vi "DAQ_DECM Configure and Measure.vi"(0 "DAQmx Tasks In":T1, 2 "Execution Option":T3, 5 "Counter Settings":T4={"Active Edge"=10280, "Duration (s)"=0.1, "Wait Type"=enum."Hardware Timed"} {"Duration (s)" format="%.2p"; "Active Edge" items=["Rising"=10280, "Falling"=10171]}, 7 "Timer - Trigger Settings":T2={"Trigger Type"=enum."No Trigger", "Digital Start Trigger Source"="", "Digital Start Trigger Edge"=10280} {"Digital Start Trigger Edge" items=["Rising"=10280, "Falling"=10171]}, 11 "error in":errorcluster) -> (4 "DAQmx Tasks Out":T1, 6 "Edge Counts":u32, 15 "error out":errorcluster)   [LabVIEW 2021, in "DAQ_Digital Edge Count Measurement.lvlib"]
doc: "Configure, initiate and fetch no of digital events/edges detected from the channel configured.\n\nNOTE: Initialize VI is recommended to create tasks instead of using tasks defined in NI-MAX directly. because initialize takes care of routing the output terminal of Timer task internally to reduce the need for additional PFI line output terminal.\n\nRefer detailed help for more details on hardware timed vs software timed digital edge counting. And use the inputs accordingly."
uses:
  DAQ_Digital Edge Count Measurement.lvlib
  Typedefs/Measurement Settings.ctl
  Typedefs/Wait Type.ctl
  Common/Typedefs/Execution Options - Measure.ctl
  Typedefs/Timer - Trigger Settings.ctl
  Typedefs/DAQmx Tasks.ctl
  <vilib>/DAQmx/read.llb/DAQmx Read (Counter U32 1Chan 1Samp).vi
  <vilib>/DAQmx/configure/trigger.llb/DAQmx Start Trigger (Digital Edge).vi
  <vilib>/DAQmx/miscellaneous.llb/DAQmx Fill In Error Info.vi
  <resource>/objmgr/daqmx.rc
panel:
  # "Inputs"
  # "Outputs"
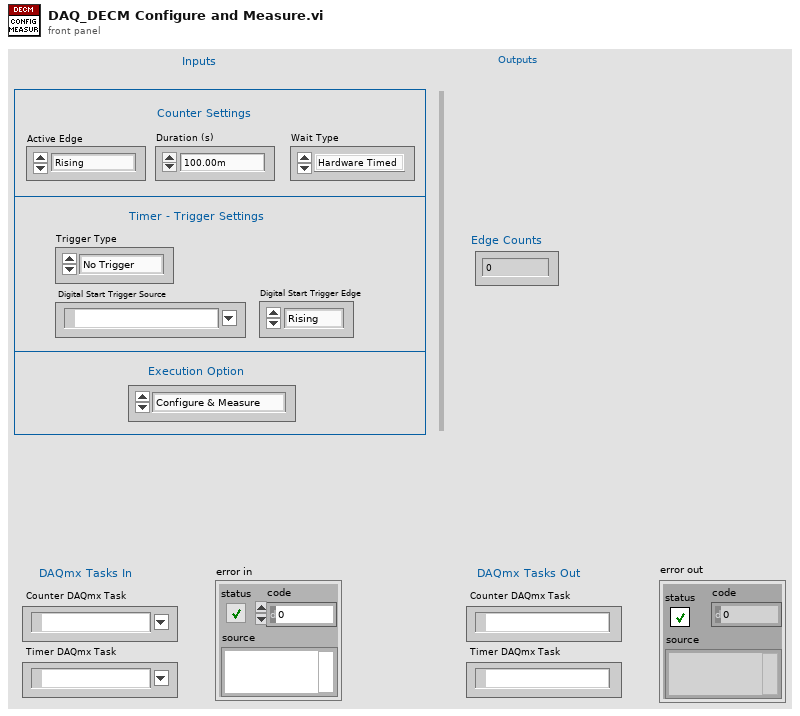
[diagram p1: front panel]
types:
  T1 = typedef "DAQ_Digital Edge Count Measurement.lvlib/DAQmx Tasks.ctl" = cluster{"Counter DAQmx Task":refnum<k21>, "Timer DAQmx Task":refnum<k21>}
  T2 = typedef "DAQ_Digital Edge Count Measurement.lvlib/Timer - Trigger Settings.ctl" = cluster{"Trigger Type":enum16{"No Trigger", "Digital Start"}, "Digital Start Trigger Source":tag, "Digital Start Trigger Edge":i32}
  T3 = typedef "Execution Options - Measure.ctl" = enum16{"Configure & Measure", "Configure only", "Measure only"}
  T4 = typedef "DAQ_Digital Edge Count Measurement.lvlib/Measurement Settings.ctl" = cluster{"Active Edge":i32, "Duration (s)":dbl, "Wait Type":T5}
  T5 = typedef "DAQ_Digital Edge Count Measurement.lvlib/Wait Type.ctl" = enum16{"Hardware Timed", "Software Timed"}
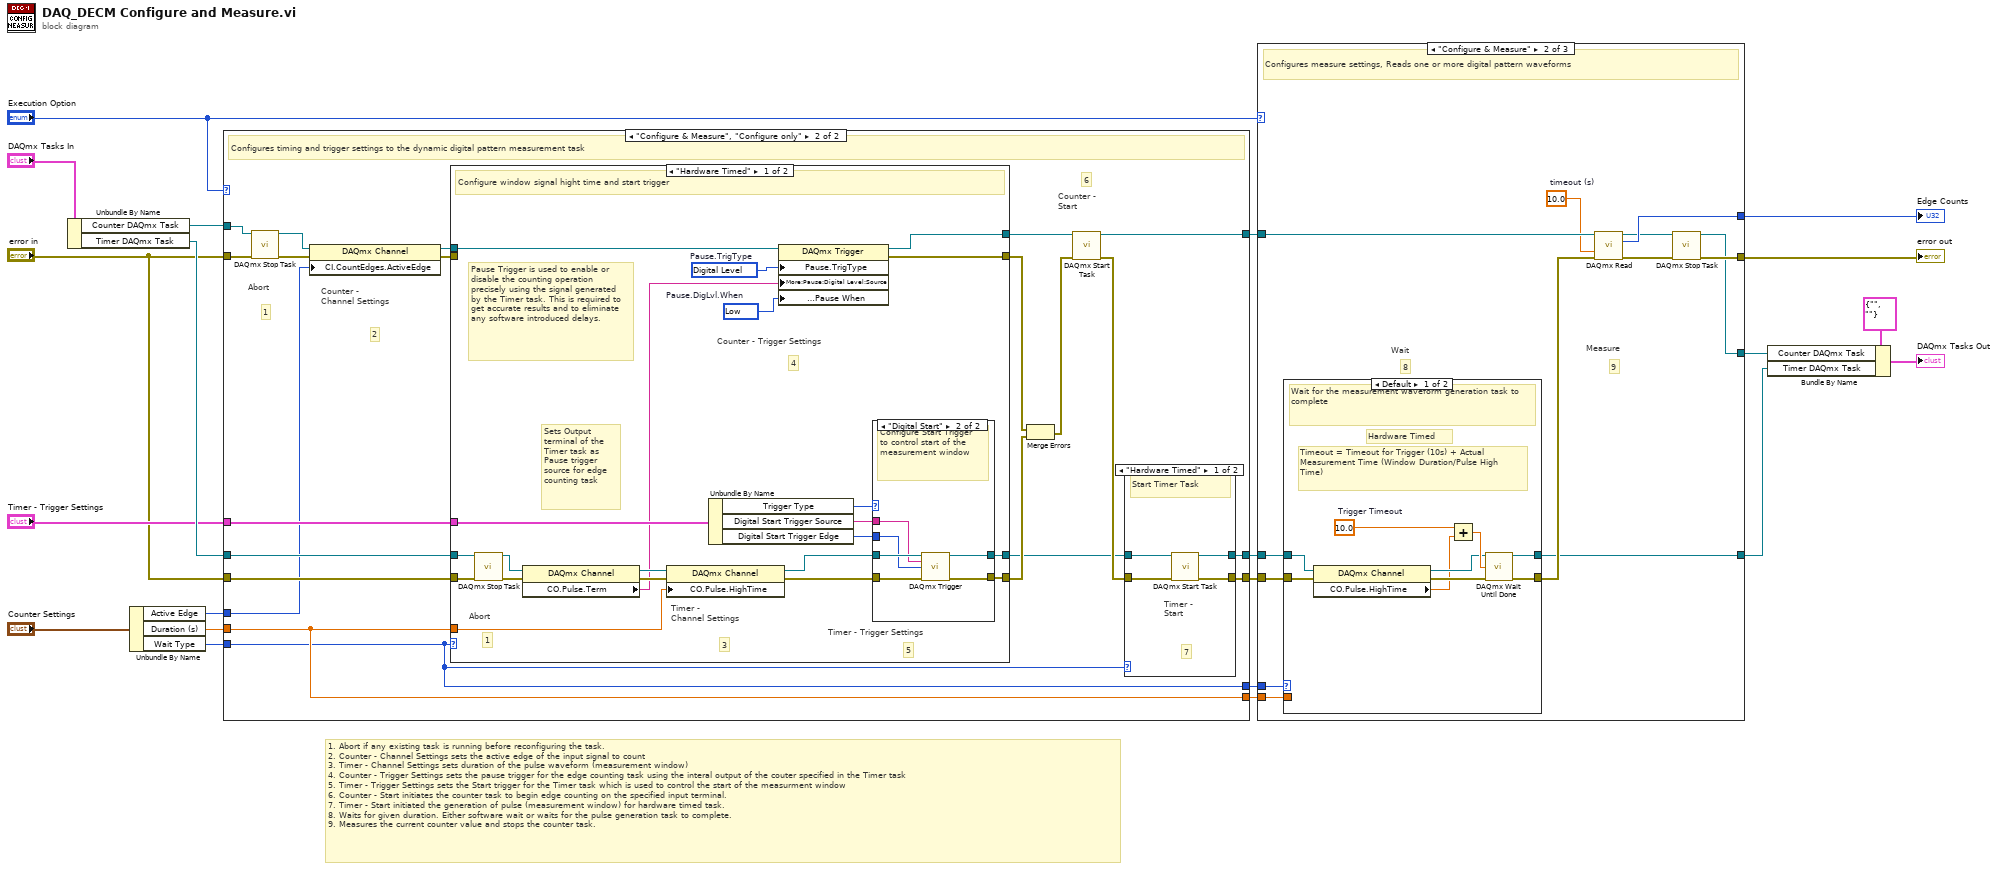
[diagram p0: block diagram]
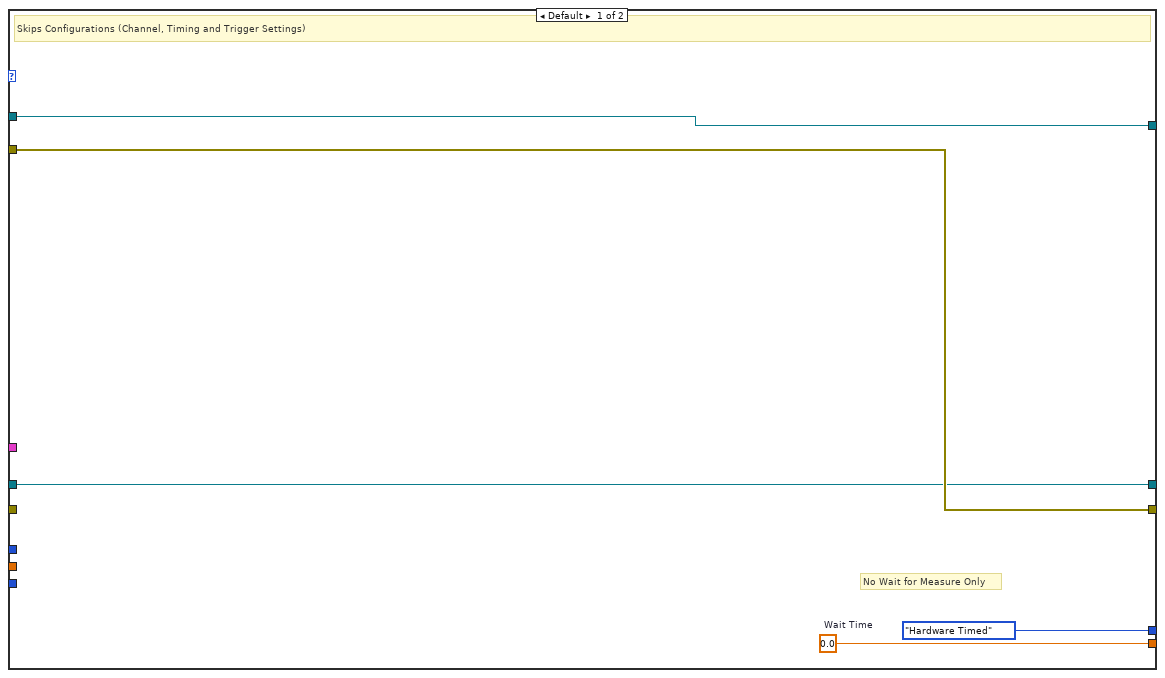
[diagram p2: hidden frame]
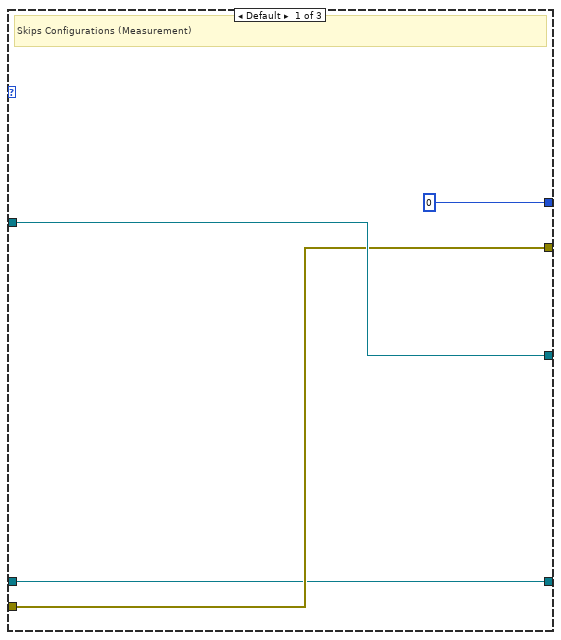
[diagram p6: hidden frame]
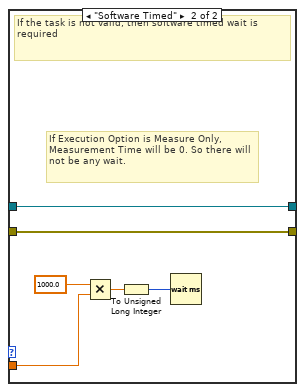
[diagram p7: hidden frame]
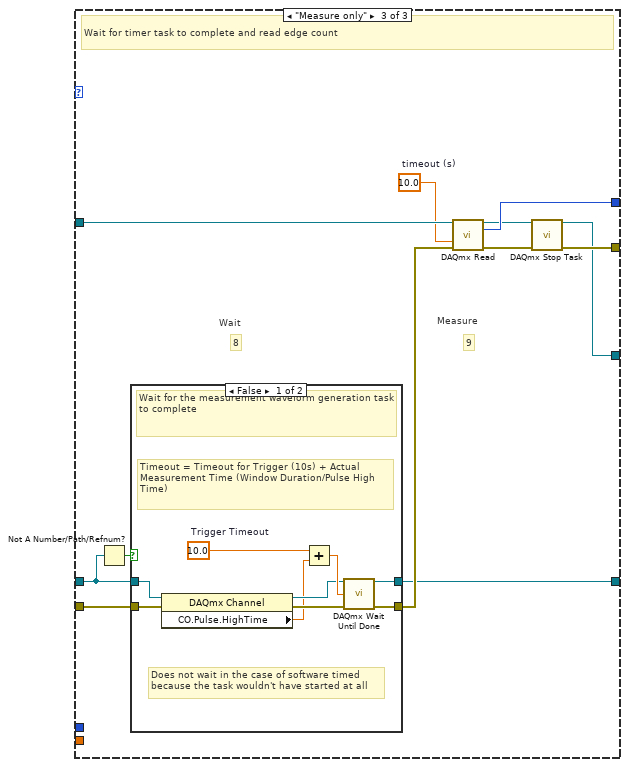
[diagram p8: hidden frame]
diagram:
  # "1. Abort if any existing task is running before reconfiguring the task.\n2. Counter - Channel Settings sets the active edge of the input signal to count\n3. Timer - Channel Settings sets duration of the pulse waveform (measurement window)\n4. Counter - Trigger Settings sets the pause trigger for the edge counting task using the interal output of the couter specified in the Timer task\n5. Timer - Trigger Settings sets the Start trigger for the Timer task which is used to control the start of the measurment window\n6. Counter - Start initiates the counter task to begin edge counting on the specified input terminal.\n7. Timer - Start initiated the generation of pulse (measurement window) for hardware timed task.\n8. Waits for given duration. Either software wait or waits for the pulse generation task to complete.\n9. Measures the current counter value and stops the counter task."
  n1 = Unbundle By Name("DAQmx Tasks In") -> ("Counter DAQmx Task"=w14:refnum<k21>, "Timer DAQmx Task"=w13:refnum<k21>)
  n2 = Unbundle By Name("Counter Settings") -> ("Active Edge"=w4:i32, "Duration (s)"=w3:dbl, "Wait Type"=w2:T5)
  n3 = case shown="\"Configure & Measure\", \"Configure only\"" "Execution Option" {
    tunnel: "error in" -> [w26 w43]
    tunnel: w14 -> [w25 w47]
    tunnel: [w25 w46] -> w20
    tunnel: [w26 w37] -> w21
    tunnel: w13 -> [w24 w30]
    tunnel: [w24 w38] -> w16
    tunnel: "Timer - Trigger Settings" -> [_ w36]
    tunnel: [w23 w28] -> w7
    tunnel: "error in" -> [_ w31]
    tunnel: w4 -> [_ w29]
    tunnel: w3 -> [_ w28]
    tunnel: w2 -> [_ w27]
    tunnel: [Wait_Type."Hardware Timed" ("Wait Type") w27] -> w1
    frame Default {
      w23 = 0.0  # Wait Time
      # "No Wait for Measure Only"
      # "Skips Configurations (Channel, Timing and Trigger Settings)"
    }
    frame "Configure & Measure", "Configure only" {
      # "6"
      # "2"
      # "1"
      # "Counter - \nStart"
      # "Counter - \nChannel Settings"
      # "Abort"
      # "Configures timing and trigger settings to the dynamic digital pattern measurement task"
      n4 = call <vilib>:"DAQmx Stop Task.vi"("task/channels in"=w47, "error in"=w43) -> ("task out"=w44:refnum<k21>, "error out"=w45:errorcluster)  [unwired: 12 in]
      n5 = property class="DAQmx Channel"(reference=w44, error in=w45, "CI.CountEdges.ActiveEdge"=w29) -> (reference out=w33:refnum<k21>, error out=w35:errorcluster)
      n6 = case shown="\"Hardware Timed\"" w27 {
        tunnel: w30 -> [w53 w79]
        tunnel: w31 -> [w67 w80]
        tunnel: w28 -> [w65 _]
        tunnel: [w64 w80] -> w42
        tunnel: [w63 w79] -> w39
        tunnel: w36 -> [w62 _]
        tunnel: w35 -> [_ w78]
        tunnel: [w56 w78] -> w34
        tunnel: w33 -> [w55 w77]
        tunnel: [w54 w77] -> w32
        frame "Hardware Timed" {
          w57 = 10214 items=["High"=10192, "Low"=10214]  # Pause.DigLvl.When
          w58 = 10152 items=["Analog Level"=10101, "Analog Window"=10103, "Digital Level"=10152, "Digital Pattern"=10398, "None"=10230]  # Pause.TrigType
          # "Pause Trigger is used to enable or disable the counting operation precisely using the signal generated by the Timer task. This is required to get accurate results and to eliminate any software introduced delays."
          # "5"
          # "4"
          # "3"
          # "Timer - \nChannel Settings"
          # "1"
          # "Abort"
          # "Sets Output terminal of the Timer task as Pause trigger source for edge counting task"
          # "Counter - Trigger Settings"
          # "Timer - Trigger Settings"
          # "Configure window signal hight time and start trigger"
          n7 = call <vilib>:"DAQmx Stop Task.vi"("task/channels in"=w53, "error in"=w67) -> ("task out"=w50:refnum<k21>, "error out"=w52:errorcluster)  [unwired: 12 in]
          n8 = property class="DAQmx Channel"(reference=w50, error in=w52) -> (reference out=w49:refnum<k21>, error out=w51:errorcluster, "CO.Pulse.Term"=w48:tag)
          n9 = property class="DAQmx Channel"(reference=w49, error in=w51, "CO.Pulse.HighTime"=w65) -> (reference out=w68:refnum<k21>, error out=w66:errorcluster)
          n10 = Unbundle By Name(w62) -> ("Trigger Type"=w61:enum16{"No Trigger", "Digital Start"}, "Digital Start Trigger Source"=w60:tag, "Digital Start Trigger Edge"=w59:i32)
          n11 = property class="DAQmx Trigger"(reference=w55, "Pause.TrigType"=w58, "More:Pause:Digital Level:Source"=w48, "More:Pause:Digital Level:Pause When"=w57) -> (reference out=w54:refnum<k21>, error out=w56:errorcluster)  [unwired: 1 in]
          n12 = case shown="\"Digital Start\"" w61 {
            tunnel: w68 -> [w70 w76]
            tunnel: w66 -> [w69 w75]
            tunnel: [w70 w73] -> w63
            tunnel: [w69 w74] -> w64
            tunnel: w60 -> [_ w72]
            tunnel: w59 -> [_ w71]
            frame Default {
              # "Skip start trigger. Pulse will be generated immediately"
            }
            frame "Digital Start" {
              # "Configure Start Trigger to control start of the measurement window"
              n13 = call-poly <vilib>:"DAQmx Trigger.vi"("task/channels in"=w76, "source"=w72, "edge"=w71, "error in"=w75) -> ("task out"=w73:refnum<k21>, "error out"=w74:errorcluster)  [unwired: 10 in]
            }
          }
        }
        frame Default {
          # "No configurations for window task"
        }
      }
      n14 = Merge Errors(w34, w42) -> (w41:errorcluster)
      n15 = call <vilib>:"DAQmx Start Task.vi"("task/channels in"=w32, "error in"=w41) -> ("task out"=w46:refnum<k21>, "error out"=w40:errorcluster)  [unwired: 12 in]
      n16 = case shown="\"Hardware Timed\"" w27 {
        tunnel: w40 -> [w84 w86]
        tunnel: w39 -> [w83 w85]
        tunnel: [w81 w86] -> w37
        tunnel: [w82 w85] -> w38
        frame "Hardware Timed" {
          # "7"
          # "Timer - \nStart"
          # "Start Timer Task"
          n17 = call <vilib>:"DAQmx Start Task.vi"("task/channels in"=w83, "error in"=w84) -> ("task out"=w82:refnum<k21>, "error out"=w81:errorcluster)  [unwired: 12 in]
        }
        frame Default {
          # "Task Invalid"
        }
      }
    }
  }
  n18 = case shown="\"Configure & Measure\"" "Execution Option" {
    tunnel: w20 -> [w90 w103 w130]
    tunnel: w21 -> [w89 w99 w126]
    tunnel: [w90 w91 w119] -> w9
    tunnel: [w89 w93 w121] -> w19
    tunnel: [u32 0 ("data") w100 w127] -> w18
    tunnel: w16 -> [w87 w95 w123]
    tunnel: w7 -> [_ w98 _]
    tunnel: [w87 w96 w124] -> w8
    tunnel: w1 -> [_ w94 _]
    frame Default {
      # "Skips Configurations (Measurement)"
    }
    frame "Configure & Measure" {
      w101 = 10.0  # timeout (s)
      # "9"
      # "8"
      # "Measure"
      # "Wait"
      # "Configures measure settings, Reads one or more digital pattern waveforms"
      n19 = case shown="Default" w94 {
        tunnel: w99 -> [w112 w114]
        tunnel: w98 -> [_ w118]
        tunnel: [w111 w114] -> w97
        tunnel: w95 -> [w104 w113]
        tunnel: [w110 w113] -> w96
        frame Default {
          w108 = 10.0  # Trigger Timeout
          # "Hardware Timed"
          # "Timeout = Timeout for Trigger (10s) + Actual Measurement Time (Window Duration/Pulse High Time)"
          # "Wait for the measurement waveform generation task to complete"
          n20 = property class="DAQmx Channel"(reference=w104, error in=w112) -> (reference out=w106:refnum<k21>, error out=w107:errorcluster, "CO.Pulse.HighTime"=w105:dbl)
          n21 = Add(x=w108, y=w105) -> (x+y=w109:dbl)
          n22 = call <vilib>:"DAQmx Wait Until Done.vi"("task/channels in"=w106, "timeout (sec)"=w109, "error in"=w107) -> ("task out"=w110:refnum<k21>, "error out"=w111:errorcluster)  [unwired: 11 in]
        }
        frame "Software Timed" {
          # "If Execution Option is Measure Only, Measurement Time will be 0. So there will not be any wait."
          # "If the task is not valid, then software timed wait is required"
          n23 = Multiply(x=1000.0, y=w118) -> (x*y=w116:dbl)
          n24 = To Unsigned Long Integer(number=w116) -> (unsigned 32bit integer=w115:u32)
          n25 = Wait (ms)(milliseconds to wait=w115) -> ()  [unwired: 1 out]
        }
      }
      n26 = call-poly <vilib>:"DAQmx Read.vi"("task/channels in"=w103, "timeout"=w101, "error in"=w97) -> ("task out"=w92:refnum<k21>, "data"=w100:u32, "error out"=w102:errorcluster)  [unwired: 10 in]
      n27 = call <vilib>:"DAQmx Stop Task.vi"("task/channels in"=w92, "error in"=w102) -> ("task out"=w91:refnum<k21>, "error out"=w93:errorcluster)  [unwired: 12 in]
    }
    frame "Measure only" {
      w128 = 10.0  # timeout (s)
      # "9"
      # "8"
      # "Measure"
      # "Wait"
      # "Wait for timer task to complete and read edge count"
      n28 = Not A Number/Path/Refnum?(number/path/refnum=w123) -> (NaN/Path/Refnum?=w122:bool)
      n29 = case shown="False" w122 {
        tunnel: w126 -> [w139 w141]
        tunnel: [w138 w141] -> w125
        tunnel: w123 -> [w131 w140]
        tunnel: [w137 w140] -> w124
        frame False {
          w135 = 10.0  # Trigger Timeout
          # "Does not wait in the case of software timed\nbecause the task wouldn't have started at all"
          # "Timeout = Timeout for Trigger (10s) + Actual Measurement Time (Window Duration/Pulse High Time)"
          # "Wait for the measurement waveform generation task to complete"
          n30 = property class="DAQmx Channel"(reference=w131, error in=w139) -> (reference out=w133:refnum<k21>, error out=w134:errorcluster, "CO.Pulse.HighTime"=w132:dbl)
          n31 = Add(x=w135, y=w132) -> (x+y=w136:dbl)
          n32 = call <vilib>:"DAQmx Wait Until Done.vi"("task/channels in"=w133, "timeout (sec)"=w136, "error in"=w134) -> ("task out"=w137:refnum<k21>, "error out"=w138:errorcluster)  [unwired: 11 in]
        }
        frame True {
          # "No wait during measure only call in software timed task"
          # "If the task is not valid, then software timed task"
        }
      }
      n33 = call-poly <vilib>:"DAQmx Read.vi"("task/channels in"=w130, "timeout"=w128, "error in"=w125) -> ("task out"=w120:refnum<k21>, "data"=w127:u32, "error out"=w129:errorcluster)  [unwired: 10 in]
      n34 = call <vilib>:"DAQmx Stop Task.vi"("task/channels in"=w120, "error in"=w129) -> ("task out"=w119:refnum<k21>, "error out"=w121:errorcluster)  [unwired: 12 in]
    }
  }
  "error out" <- w19
  "Edge Counts" <- w18
  n35 = Bundle By Name(cluster=T1 {"Counter DAQmx Task"="", "Timer DAQmx Task"=""} ("DAQmx Tasks Out"), "Counter DAQmx Task"=w9, "Timer DAQmx Task"=w8) -> (→"DAQmx Tasks Out":T1)
